vi "snakeStep.vi"(6 "Movement":T1, 8 "error in (no error)":errorcluster, 9 "PreviousY":i32=5, 10 "PreviousX":i32=5, 11 "Snake in":refnum<class "Snake.lvclass">) -> (0 "error out":errorcluster, 1 "NextY":i32=5, 2 "NextX":i32=5, 3 "Snake out":refnum<class "Snake.lvclass">)   [LabVIEW 2014, in "Snake.lvclass"]
uses:
  Snake.lvclass
  TypeDefs/SnakeMovements.ctl
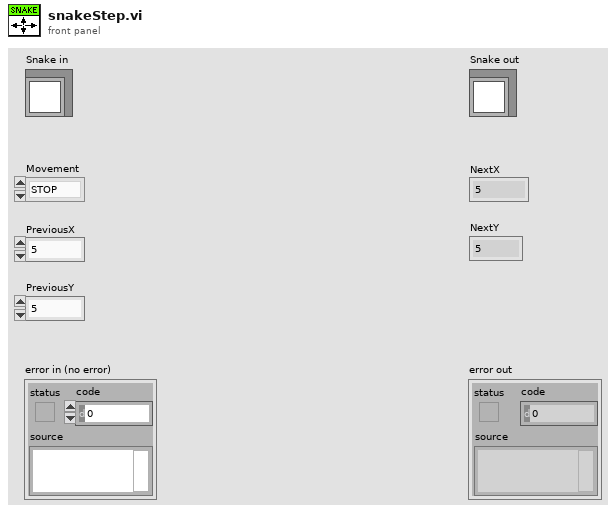
[diagram p1: front panel]
types:
  T1 = typedef "SnakeMovements.ctl" = enum16{"STOP", "UP", "DOWN", "RIGHT", "LEFT"}
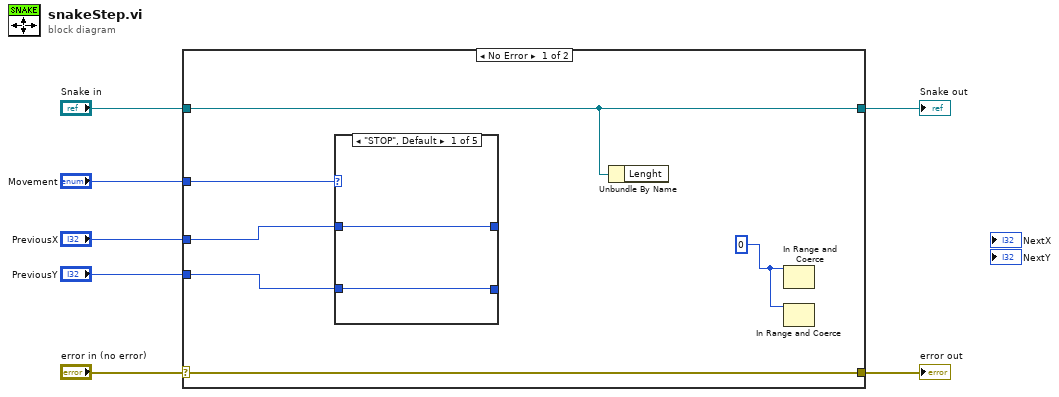
[diagram p0: block diagram]
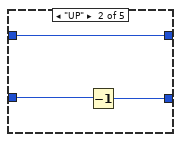
[diagram p2: hidden frame]
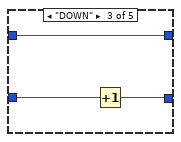
[diagram p3: hidden frame]
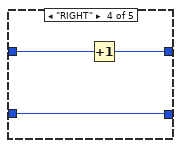
[diagram p4: hidden frame]
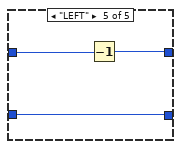
[diagram p5: hidden frame]
diagram:
  n1 = case shown="No Error" "error in (no error)" {
    selector: "error in (no error)" -> [w17 w33]
    tunnel: [w17 w33] -> w6
    tunnel: [w8 w32] -> w4
    tunnel: "Snake in" -> [w8 w32]
    tunnel: "Movement" -> [w11 _]
    tunnel: "PreviousX" -> [w10 _]
    tunnel: "PreviousY" -> [w9 _]
    frame No Error {
      w14 = 0 ("upper limit")
      n2 = case shown="\"STOP\", Default" w11 {
        tunnel: w10 -> [w19 w20 w23 w28 w31]
        tunnel: w9 -> [w18 w22 w25 w27 w29]
        tunnel: [w18 w21 w24 w27 w29] -> _
        tunnel: [w19 w20 w23 w26 w30] -> _
        frame "STOP", Default {
        }
        frame "UP" {
          n3 = Decrement(x=w22) -> (x-1=w21:i32)
        }
        frame "DOWN" {
          n4 = Increment(x=w25) -> (x+1=w24:i32)
        }
        frame "RIGHT" {
          n5 = Increment(x=w28) -> (x+1=w26:i32)
        }
        frame "LEFT" {
          n6 = Decrement(x=w31) -> (x-1=w30:i32)
        }
      }
      n7 = Unbundle By Name(w8) -> ()  [unwired: 1 out]
      n8 = In Range and Coerce(upper limit=w14) -> (x=w16:i32, lower limit=w12:i32)  [unwired: 2 out]
      n9 = In Range and Coerce(upper limit=w14) -> (x=w15:i32, lower limit=w13:i32)  [unwired: 2 out]
    }
    frame Error {
    }
  }
  "error out" <- w6
  "Snake out" <- w4
